vi "InitXYGraph.vi"(8 "error in (no error)":errorcluster, 11 "XYGraph in":refnum<vi>) -> (0 "error out":errorcluster, 3 "XYGraph out":refnum<vi>)   [LabVIEW 2023]
doc: "Initializes xygraph control"
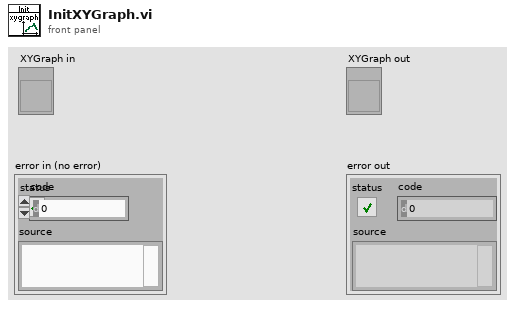
[diagram p1: front panel]
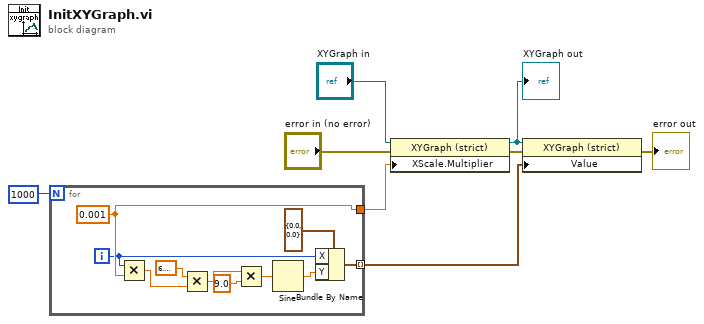
[diagram p0: block diagram]
diagram:
  n1 = for {
    N: 1000 -> [_]
    tunnel: [w18] -> w8 mode=indexing
    tunnel: [w15] -> w6
    i -> [w14]
    w15 = 0.001 ("y")
    n2 = Multiply(x=w14, y=w15) -> (x*y=w13:dbl)
    n3 = Multiply(x=6.283185307179586, y=w13) -> (x*y=w11:dbl)
    n4 = Multiply(x=w11, y=9.0) -> (x*y=w9:dbl)
    n5 = Sine(x=w9) -> (sin(x)=w16:dbl)
    n6 = Bundle By Name(cluster=cluster{"X":dbl, "Y":dbl} {"X"=0.0, "Y"=0.0}, "X"=w14, "Y"=w16) -> (w18:cluster{"X":dbl, "Y":dbl})
  }
  n7 = property class="XYGraph (strict)"(reference="XYGraph in", error in="error in (no error)", "XScale.Multiplier"=w6) -> (reference out=w7:refnum<vi>, error out=w3:errorcluster)
  "XYGraph out" <- w7
  n8 = property class="XYGraph (strict)"(reference=w7, error in=w3, "Value"=w8) -> (error out=→"error out":errorcluster)  [unwired: 1 out]
